vi "Calculation average reflectance Batch.vi"(1 "保存路径":path, 2 "file path (dialog if empty)":path=path "F:/fh/传输D/2015谷粒实验/提取数据/原始总反射率/1-原始总反射率txt") -> ()   [LabVIEW 2015]
panel:
  out "filenames":string[](array[string])
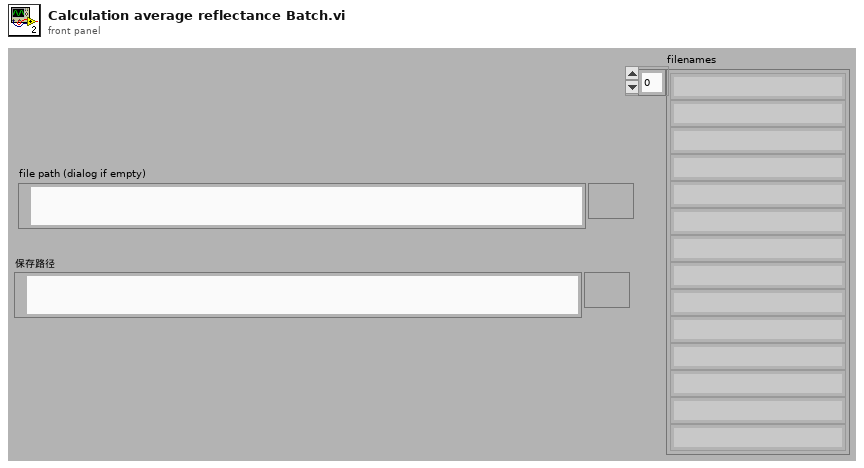
[diagram p1: front panel]
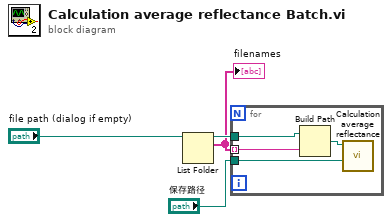
[diagram p0: block diagram]
diagram:
  n1 = List Folder(path="file path (dialog if empty)") -> (path out=w3:path, filenames=w2:string[])  [unwired: 1 in, 4 out]
  "filenames" <- w2
  n2 = for {
    tunnel: w3 -> [w8]
    tunnel: w2 -> [w7] mode=indexing
    tunnel: "保存路径" -> [w5]
    n3 = Build Path(base path=w8, name or relative path=w7) -> (appended path=w6:path)
    n4 = call "Calculation average reflectance.vi"("保存路径"=w5, "file path (dialog if empty)"=w6) -> ()  [unwired: 10 out]
  }
